vi "LSet.vi"(0 "reference in":refnum<class "Redis.lvclass">, 1 "Key":string, 7 "Index":i32, 9 "Element":string, 11 "Error In":errorcluster) -> (4 "reference out":refnum<class "Redis.lvclass">, 8 "String":string, 15 "Error Out":errorcluster)   [LabVIEW 2020, in "Redis.lvclass"]
doc: "<b>LSET</b>\n\nSets the list element at index to element. For more information on the index argument, see LINDEX.\n\nAn error is returned for out of range indexes."
uses:
  Redis.lvclass
  Redis.lvclass/Redis.ctl
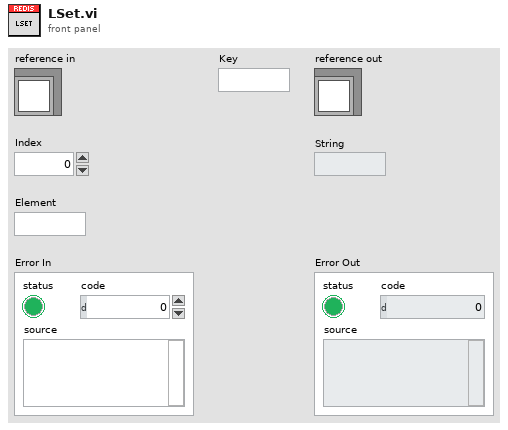
[diagram p1: front panel]
types:
  T1 = typedef "Redis.lvclass/RedisDataType.ctl" = cluster{"Reply Type":T2, "Integer":i64, "String":string, "Multibulk":variant[], "StringData":string[]}
  T2 = typedef "Redis.lvclass/ReplyDataTypeEnum.ctl" = enum16{"None", "Error", "Status", "Nil", "Integer", "String", "Multibulk"}
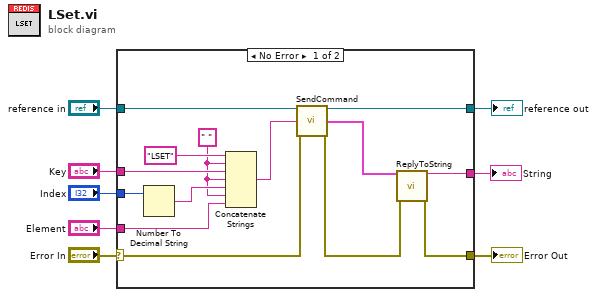
[diagram p0: block diagram]
diagram:
  n1 = case shown="No Error" "Error In" {
    selector: "Error In" -> [w20 w24]
    tunnel: [w11 w24] -> w7
    tunnel: [w22 w23] -> w5
    tunnel: "reference in" -> [w21 w23]
    tunnel: "Key" -> [w18 _]
    tunnel: "Index" -> [w16 _]
    tunnel: "Element" -> [w13 _]
    tunnel: [w9 _] -> w1
    frame No Error {
      w14 = " "
      n2 = Number To Decimal String(number=w16) -> (decimal integer string=w15:string)  [unwired: 1 in]
      n3 = Concatenate Strings("LSET", w14, w18, w14, w15, w14, w13) -> (w17:string)
      n4 = call "SendCommand.vi"("reference in"=w21, "Command"=w17, "Error In"=w20) -> ("reference out"=w22:refnum<class "Redis.lvclass">, "Data"=w10:T1, "Error Out"=w12:errorcluster)  [unwired: 10 in]
      n5 = call "ReplyToString.vi"("Reply"=w10, "Error In"=w12) -> ("String"=w9:string, "Error Out"=w11:errorcluster)  [unwired: 12 in]
    }
    frame Error {
    }
  }
  "Error Out" <- w7
  "reference out" <- w5
  "String" <- w1
